vi "ArdnoString2Array.vi"(9 "Valve (A1-C8),\n comma separated":string, 11 "Array in":bool[](array[boolean])) -> (3 "Array out":bool[](array[boolean]))   [LabVIEW 2018]
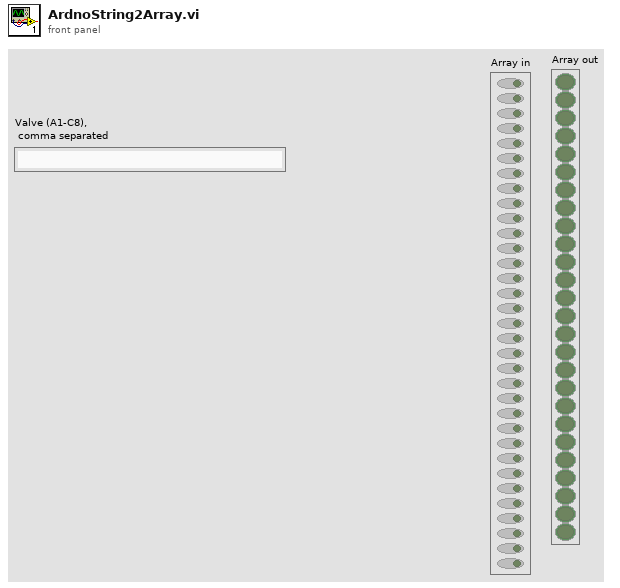
[diagram p1: front panel]
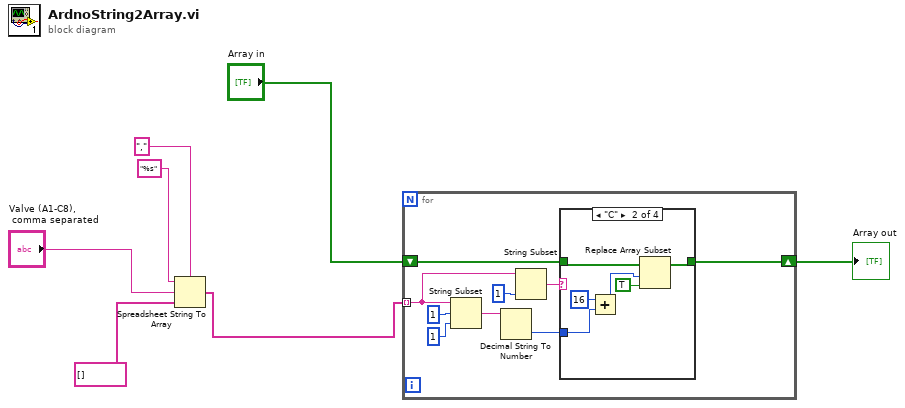
[diagram p0: block diagram]
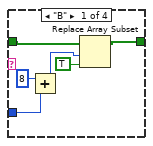
[diagram p2: hidden frame]
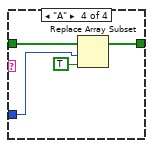
[diagram p4: hidden frame]
diagram:
  n1 = Spreadsheet String To Array(delimiter (Tab)=",", format string="%s", spreadsheet string="Valve (A1-C8),\n comma separated", array type (2D Dbl)=string[] []) -> (array=w4:string[])
  n2 = for {
    tunnel: w4 -> [w13] mode=indexing
    shift-right: [w8] -> w2
    shift-left: "Array in" -> [w9]
    n3 = String Subset(string=w13, offset (0)=1, length (rest)=1 ("length (rest)")) -> (substring=w11:string)
    n4 = Decimal String To Number(string=w11) -> (number=w10:i32)  [unwired: 2 in, 1 out]
    n5 = String Subset(string=w13, length (rest)=1 ("length (rest)")) -> (substring=w15:string)  [unwired: 1 in]
    n6 = case shown="\"C\"" w15 {
      tunnel: w10 -> [w19 w23 _ w32]
      tunnel: w9 -> [w21 w24 w29 w33]
      tunnel: [w20 w25 w29 w30] -> w8
      frame "B" {
        n7 = Add(x=8, y=w19) -> (x+y=w18:i32)
        n8 = Replace Array Subset(array=w21, new element=TRUE ("new element/subarray"), index=w18) -> (w20:bool[])
      }
      frame "C" {
        n9 = Add(x=16, y=w23) -> (x+y=w27:i32)
        n10 = Replace Array Subset(array=w24, new element=TRUE ("new element/subarray"), index=w27) -> (w25:bool[])
      }
      frame Default {
      }
      frame "A" {
        n11 = Replace Array Subset(array=w33, new element=TRUE ("new element/subarray"), index=w32) -> (w30:bool[])
      }
    }
  }
  "Array out" <- w2
